vi "Custom Four Motor Drive Configure.vi"(0 "timeout (s)":dbl=0.1, 2 "Rear Right":T2, 3 "Front Right":T2, 8 "Safety Config State":T1, 9 "Invert Right Side?":bool=TRUE, 10 "Rear Left":T2, 11 "Front Left":T2) -> ()   [LabVIEW 2012]
uses:
  <vilib>/Rock Robotics/SystemInterfaces/DIO/FPGA_DIOPWMChannel.ctl
  <vilib>/Rock Robotics/WPI/SafetyOutput/WPI_SafetyOutputConfigMenu.ctl
  <vilib>/Rock Robotics/WPI/MotorControl/WPI_MotorControlOpen Talon.vi
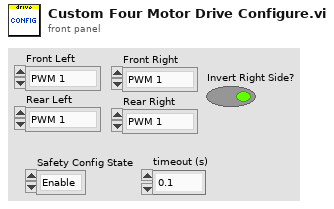
[diagram p1: front panel]
types:
  T1 = typedef "WPI_SafetyOutputConfigMenu.ctl" = enum16{"Enable", "Disable"}
  T2 = typedef "FPGA_DIOPWMChannel.ctl" = enum8{"PWM 1", "PWM 2", "PWM 3", "PWM 4", "PWM 5", "PWM 6", "PWM 7", "PWM 8", "PWM 9", "PWM 10", "Invalid"}
  T3 = typedef "WPI_MotorControlDeviceRef.ctl" = cluster{"DeviceStatus":errorcluster, "Type":enum16{"PWM", "CAN"}, "PWM":cluster{"Digital Module":T4, "PWM Channel":T2, "DeadBand":T5}, "CAN":cluster{"Device Number":u8, "Control Mode":T6, "Semaphore":T7, "Max Vout":dbl}, "Invert":bool, "TransformRef":T8, "InvTransformRef":T8}
  T4 = typedef "FPGA_TypedefDigitalModule.ctl" = enum16{"Digital Module 1", "Digital Module 2"}
  T5 = typedef "WPI_PWMDeadband.ctl" = cluster{"Name":string, "maxPositivePwm":i32, "minPositivePwm":i32, "centerPwm":i32, "maxNegativePwm":i32, "minNegativePwm":i32, "angularRange":u16}
  T6 = typedef "WPI_CANJaguar_ControlMode.ctl" = enum8{"Percent VBus", "Current", "Speed", "Position", "Voltage"}
  T7 = typedef "Semaphore RefNum" = refnum<k1>
  T8 = typedef "WPI_PWMTransform_ConPane.ctl" = refnum<vi>
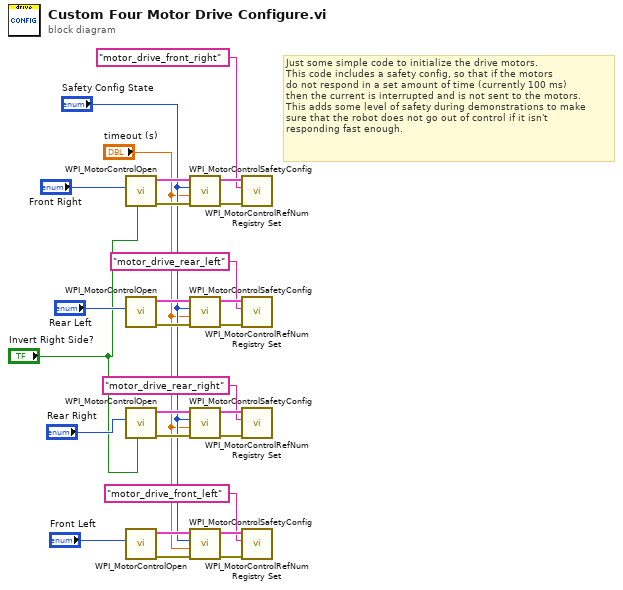
[diagram p0: block diagram]
diagram:
  # "Just some simple code to initialize the drive motors. \nThis code includes a safety config, so that if the motors\ndo not respond in a set amount of time (currently 100 ms) \nthen the current is interrupted and is not sent to the motors.\nThis adds some level of safety during demonstrations to make\nsure that the robot does not go out of control if it isn't \nresponding fast enough."
  n1 = call-poly <vilib>:"WPI_MotorControlOpen.vi"("Invert"="Invert Right Side?", "PWM Channel"="Front Right") -> ("error out"=w12:errorcluster, "MotorControlDeviceRef"=w13:T3)  [unwired: 8 in]
  n2 = call-poly <vilib>:"WPI_MotorControlOpen.vi"("PWM Channel"="Rear Left") -> ("error out"=w19:errorcluster, "MotorControlDeviceRef"=w18:T3)  [unwired: 9 in]
  n3 = call-poly <vilib>:"WPI_MotorControlOpen.vi"("Invert"="Invert Right Side?", "PWM Channel"="Rear Right") -> ("error out"=w27:errorcluster, "MotorControlDeviceRef"=w26:T3)  [unwired: 8 in]
  n4 = call-poly <vilib>:"WPI_MotorControlOpen.vi"("PWM Channel"="Front Left") -> ("error out"=w20:errorcluster, "MotorControlDeviceRef"=w21:T3)  [unwired: 9 in]
  n5 = call <vilib>:"WPI_MotorControlSafetyConfig.vi"("error in (no error)"=w12, "timeout (s)"="timeout (s)", "mode"="Safety Config State", "MotorControlDevRef"=w13) -> ("error out"=w14:errorcluster, "MotorControlDevRef"=w15:T3)  [unwired: 6 in]
  n6 = call <vilib>:"WPI_MotorControlSafetyConfig.vi"("error in (no error)"=w19, "timeout (s)"="timeout (s)", "mode"="Safety Config State", "MotorControlDevRef"=w18) -> ("error out"=w17:errorcluster, "MotorControlDevRef"=w16:T3)  [unwired: 6 in]
  n7 = call <vilib>:"WPI_MotorControlSafetyConfig.vi"("error in (no error)"=w27, "timeout (s)"="timeout (s)", "mode"="Safety Config State", "MotorControlDevRef"=w26) -> ("error out"=w25:errorcluster, "MotorControlDevRef"=w24:T3)  [unwired: 6 in]
  n8 = call <vilib>:"WPI_MotorControlSafetyConfig.vi"("error in (no error)"=w20, "timeout (s)"="timeout (s)", "mode"="Safety Config State", "MotorControlDevRef"=w21) -> ("error out"=w22:errorcluster, "MotorControlDevRef"=w23:T3)  [unwired: 6 in]
  n9 = call <vilib>:"WPI_MotorControlRefNum Registry Set.vi"("error in (no error)"=w14, "refnum name"="motor_drive_front_right", "MotorControlDevRef"=w15) -> ()  [unwired: 7 in, 2 out]
  n10 = call <vilib>:"WPI_MotorControlRefNum Registry Set.vi"("error in (no error)"=w17, "refnum name"="motor_drive_rear_left", "MotorControlDevRef"=w16) -> ()  [unwired: 7 in, 2 out]
  n11 = call <vilib>:"WPI_MotorControlRefNum Registry Set.vi"("error in (no error)"=w25, "refnum name"="motor_drive_rear_right", "MotorControlDevRef"=w24) -> ()  [unwired: 7 in, 2 out]
  n12 = call <vilib>:"WPI_MotorControlRefNum Registry Set.vi"("error in (no error)"=w22, "refnum name"="motor_drive_front_left", "MotorControlDevRef"=w23) -> ()  [unwired: 7 in, 2 out]
